vi "TXRX 5785 No DDC Measure Phase Stability_AI AO TCLK.vi"() -> ()   [LabVIEW 2019]
uses:
  <vilib>/userDefined/High Color/nirio_resource_hc.ctl
  <instrlib>/FlexRIO/API/Host/v1/NI FlexRIO/API/Reference Clock Source.ctl
  <vilib>/Analysis/1siggen.llb/Ramp Pattern by Delta.vi
  <instrlib>/FlexRIO/API/Host/v1/NI FlexRIO/API/Configure Reference Clock.vi
  <instrlib>/FlexRIO/API/Host/v1/NI FlexRIO/API/Get Property Reference - Fpga Small.vi
  <instrlib>/FlexRIO/API/Host/v1/NI FlexRIO/API/Configure Immediate Start Trigger.vi
  <instrlib>/FlexRIO/API/Host/v1/NI FlexRIO/API/Configure Digital Edge Start Trigger.vi
  <instrlib>/FlexRIO/API/Host/v1/NI FlexRIO/API/Read Stream 1D WDT.vi
  <vilib>/measure/matone.llb/Extract Single Tone Information N Chan.vi
  <vilib>/FPGAPlugInAG/Dynamic/niLvFpga_Close_Dynamic.vi
  <vilib>/Utility/file.llb/Write Delimited Spreadsheet (DBL).vi
  <vilib>/rvi/interface/nirviCloseFPGA/nirviCloseFPGA.xnode
  <vilib>/measure/NI_MAPro.lvlib
  <vilib>/Analysis/NI_AALPro.lvlib
  <vilib>/Analysis/NI_AALBase.lvlib
  <instrlib>/FlexRIO/API/Host/v1/NI FlexRIO API v1.lvlib
  <resource>/objmgr/niflexrioapiStream.rc
  Common/Original 5785 Example/Host/GettingStarted_5785_Host.lvlib
  <resource>/objmgr/niflexrioapiTrigger.rc
panel:
  out "read data 2":waveform(dbl)[](graph)=[{"t0"=timestamp(0 s since 1904-01-01), "dt"=3.125e-10, "Y"=[]}, {"t0"=timestamp(0 s since 1904-01-01), "dt"=3.125e-10, "Y"=[]}, {"t0"=timestamp(0 s since 1904-01-01), "dt"=3.125e-10, "Y"=[]}, {"t0"=timestamp(0 s since 1904-01-01), "dt"=3.125e-10, "Y"=[]}]
  in  "ABORT":bool
  in  "flexrio tranceivers":T2(array[cluster])
  out "error out":errorcluster
  out "read data":waveform(dbl)[](graph)=[{"t0"=timestamp(0 s since 1904-01-01), "dt"=3.125e-10, "Y"=[]}, {"t0"=timestamp(0 s since 1904-01-01), "dt"=3.125e-10, "Y"=[]}, {"t0"=timestamp(0 s since 1904-01-01), "dt"=3.125e-10, "Y"=[]}, {"t0"=timestamp(0 s since 1904-01-01), "dt"=3.125e-10, "Y"=[]}]
  in  "samples to acquire":u64=65536
  out "Output Waveform":waveform(dbl)[](graph)
  in  "sampling info":cluster{"Fs":dbl, "#s":dbl}={"Fs"=3200000000.0, "#s"=1600.0}
  in  "amplitude":dbl=0.2 format="%#_13p"
  in  "frequency":dbl=32000000.0 format="%0.2p"
  in  "trigger mode":enum16{"Immediate", "Digital"}(ring)
  in  "trigger source":string(combo)
  out "error out 2":errorcluster
  out "Results":T3(array[cluster])=[{"frequency (Hz)"=10000000.0, "mean skew"=-8.648150356036804e-11, "skew std dev"=2.4099744101288974e-11, "skew pk-pk"=7.257205272197028e-11, "skews"=[-7.634263492782065e-11, -5.206006966613256e-11, -7.567203753755032e-11, -1.2206425690719055e-10, -8.304777374940357e-11, -1.0474159284040468e-10, -9.611917176930304e-11, -4.9492204185220274e-11, -9.19555565839358e-11, -1.1331973743671892e-10]}, {"frequency (Hz)"=50000000.0, "mean skew"=-3.785636387258172e-12, "skew std dev"=7.66796131206532e-12, "skew pk-pk"=2.0450056958183634e-11, "skews"=[-1.4356702041335054e-11, -1.6858595580753508e-11, 3.9640356991197555e-13, 2.1898804487920657e-12, 3.591461377430126e-12, 5.627769488312176e-13, 2.0778793414142268e-12, -9.498878640875245e-13, -2.082260920467761e-12, -1.242731915231749e-11]}, {"frequency (Hz)"=100000000.0, "mean skew"=2.9756926970137243e-12, "skew std dev"=4.126438485430937e-12, "skew pk-pk"=1.3178656356672357e-11, "skews"=[-3.803864807523877e-12, 1.2229613162477112e-12, 3.353001868594509e-13, 6.147451569656316e-12, 3.467389040439413e-12, 9.37479154914848e-12, 3.130954906117878e-13, 5.3691066005407156e-12, 7.679194212684065e-12, -3.484981885268205e-13]}, {"frequency (Hz)"=150000000.0, "mean skew"=-3.1256285003637117e-12, "skew std dev"=2.50792505062644e-12, "skew pk-pk"=8.984925023293429e-12, "skews"=[-4.502762861812405e-12, -1.6045172273490561e-12, -2.9190171390647476e-12, -3.070990694678064e-13, -8.33215064320321e-12, -4.242400597204465e-12, -4.000839777166906e-12, 6.527743800902194e-13, -3.7005805394824356e-12, -2.2996915289763056e-12]}, {"frequency (Hz)"=200000000.0, "mean skew"=-8.350958023237677e-12, "skew std dev"=2.5975389756296594e-12, "skew pk-pk"=9.251979822405072e-12, "skews"=[-8.992508817543144e-12, -7.361526314260884e-12, -5.409418265633645e-12, -6.808722347470321e-12, -7.136097246425896e-12, -1.4661398088038717e-11, -1.0459370862648973e-11, -7.417267998914027e-12, -8.20329760295492e-12, -7.05997268848624e-12]}, {"frequency (Hz)"=250000000.0, "mean skew"=-6.229423609785982e-12, "skew std dev"=1.1181109842334413e-12, "skew pk-pk"=3.697563683201574e-12, "skews"=[-6.543472598258066e-12, -6.423877782336823e-12, -7.33916505767155e-12, -5.048427489200302e-12, -6.3111029457941555e-12, -6.605254632098134e-12, -6.962233060771497e-12, -3.95708736948471e-12, -5.448964109558302e-12, -7.654651052686284e-12]}, {"frequency (Hz)"=300000000.0, "mean skew"=-6.136089114075028e-12, "skew std dev"=9.42262857424596e-13, "skew pk-pk"=3.206385053636777e-12, "skews"=[-7.001117375279714e-12, -5.596228282724161e-12, -7.790788409887583e-12, -6.640956435014748e-12, -6.510029213872093e-12, -4.584403356250806e-12, -5.788671870420912e-12, -5.481861597872109e-12, -6.621852735719958e-12, -5.3449818637081885e-12]}, {"frequency (Hz)"=350000000.0, "mean skew"=-7.543098180047223e-12, "skew std dev"=3.8486735494540495e-13, "skew pk-pk"=1.2874637805991694e-12, "skews"=[-7.488662007824413e-12, -7.345064850347847e-12, -7.363173973336141e-12, -7.991225504656965e-12, -7.35831616172544e-12, -8.080201975318365e-12, -7.949579206730948e-12, -7.588239975011586e-12, -6.7927381947191955e-12, -7.473779950801325e-12]}, {"frequency (Hz)"=400000000.0, "mean skew"=-8.039336411333349e-12, "skew std dev"=7.425609882339821e-13, "skew pk-pk"=2.2738072930854095e-12, "skews"=[-7.656827769683663e-12, -9.457825738470782e-12, -7.679147937131138e-12, -7.995928800206408e-12, -8.83385230395903e-12, -7.54257226646767e-12, -7.31361750761873e-12, -7.184018445385372e-12, -7.962031171009181e-12, -8.767542173401512e-12]}, {"frequency (Hz)"=450000000.0, "mean skew"=-7.93200988579298e-12, "skew std dev"=7.97455496904726e-13, "skew pk-pk"=2.6238656725690157e-12, "skews"=[-7.898237136846618e-12, -8.55120393482239e-12, -8.79911402833156e-12, -7.812476697854857e-12, -7.693964239880247e-12, -6.482757646206027e-12, -8.3933125130091e-12, -9.106623318775042e-12, -7.260055680055343e-12, -7.322353662148608e-12]}, {"frequency (Hz)"=500000000.0, "mean skew"=-7.67982756908766e-12, "skew std dev"=6.672272359581462e-13, "skew pk-pk"=2.0371763701039724e-12, "skews"=[-8.507074422893644e-12, -7.0880582107488455e-12, -7.782804612094616e-12, -7.582126885479152e-12, -7.256810103118096e-12, -8.96121612129985e-12, -7.2605372159962215e-12, -7.281199578354681e-12, -6.924039751195878e-12, -8.154408789695609e-12]}, {"frequency (Hz)"=550000000.0, "mean skew"=-7.497637800191673e-12, "skew std dev"=7.103834430343908e-13, "skew pk-pk"=2.273387428636986e-12, "skews"=[-6.788566760330353e-12, -7.618981619747259e-12, -8.146972324445106e-12, -7.622320471598431e-12, -6.408580300349553e-12, -7.095092352672633e-12, -7.963135085088087e-12, -8.681967728986539e-12, -7.854698807254544e-12, -6.796062551444227e-12]}, {"frequency (Hz)"=600000000.0, "mean skew"=-6.656473926831814e-12, "skew std dev"=6.694881342261218e-13, "skew pk-pk"=1.9961300493555487e-12, "skews"=[-5.544977406952426e-12, -7.505826199727893e-12, -6.130703962050041e-12, -6.202863013065509e-12, -6.968667303110993e-12, -7.203039184312062e-12, -6.6392992458656125e-12, -6.0278794692841194e-12, -6.800376027641509e-12, -7.541107456307974e-12]}, {"frequency (Hz)"=650000000.0, "mean skew"=-6.170836312403341e-12, "skew std dev"=6.619061413781283e-13, "skew pk-pk"=2.2437727341724404e-12, "skews"=[-5.6761371841019825e-12, -6.355813112635683e-12, -5.813528117360099e-12, -5.8323315333927895e-12, -6.992345927519065e-12, -6.404883995266873e-12, -6.792134783464002e-12, -6.572966737937676e-12, -4.7485731933466245e-12, -6.5196485390086175e-12]}, {"frequency (Hz)"=700000000.0, "mean skew"=-6.189182831668323e-12, "skew std dev"=1.7157996931343636e-13, "skew pk-pk"=5.374178601958277e-13, "skews"=[-6.141615985942628e-12, -6.4858404095071854e-12, -6.233773633306086e-12, -6.2514132085703466e-12, -5.98652075251154e-12, -6.120870770642584e-12, -6.325272720314335e-12, -5.948422549311358e-12, -6.046719279911735e-12, -6.351379006665432e-12]}, {"frequency (Hz)"=750000000.0, "mean skew"=-6.5871572160487534e-12, "skew std dev"=4.41835545476434e-13, "skew pk-pk"=1.3482286990633495e-12, "skews"=[-6.408185337335485e-12, -6.6984014567953855e-12, -5.8037511563193215e-12, -5.956322167651966e-12, -6.385471028720583e-12, -7.009944685195322e-12, -6.796395481232521e-12, -6.839548682157055e-12, -6.821572309697221e-12, -7.151979855382671e-12]}, {"frequency (Hz)"=800000000.0, "mean skew"=-6.318415408299373e-12, "skew std dev"=5.360678898648873e-13, "skew pk-pk"=1.3845512042933417e-12, "skews"=[-6.991605843987897e-12, -6.471917002931961e-12, -5.868508226304447e-12, -6.587798178445769e-12, -5.6267669909771774e-12, -6.078767737351072e-12, -5.619707707506443e-12, -7.0042589117997844e-12, -6.851992861208232e-12, -6.082830622480952e-12]}, {"frequency (Hz)"=850000000.0, "mean skew"=-6.0180248346099665e-12, "skew std dev"=3.591713662163337e-13, "skew pk-pk"=1.1349470370084415e-12, "skews"=[-5.778738385130886e-12, -5.507329414754426e-12, -6.00610567960471e-12, -6.351181258112003e-12, -6.642276451762867e-12, -6.120739453272636e-12, -5.830550574804746e-12, -6.130742822105978e-12, -6.26599539616416e-12, -5.5465889103872445e-12]}, {"frequency (Hz)"=900000000.0, "mean skew"=-6.105366074378527e-12, "skew std dev"=2.6415729684293626e-13, "skew pk-pk"=9.150989335434855e-13, "skews"=[-6.100624138292147e-12, -6.176574316377945e-12, -6.247087188419655e-12, -6.696716487837525e-12, -5.835346835163569e-12, -5.994420432808338e-12, -6.201485877561482e-12, -5.78161755429404e-12, -5.8764077856967975e-12, -6.143380127333783e-12]}, {"frequency (Hz)"=950000000.0, "mean skew"=-6.431589636547766e-12, "skew std dev"=2.1126924807836585e-13, "skew pk-pk"=6.684732217835237e-13, "skews"=[-6.4527930268702555e-12, -6.67300399028584e-12, -6.020076613990734e-12, -6.561072065807103e-12, -6.250560131333176e-12, -6.440878292553848e-12, -6.404316276846632e-12, -6.580400983912426e-12, -6.244245148103377e-12, -6.6885498357742574e-12]}, {"frequency (Hz)"=1000000000.0, "mean skew"=-6.675839066411157e-12, "skew std dev"=3.266749368738765e-13, "skew pk-pk"=9.515417562958724e-13, "skews"=[-6.645668230188316e-12, -7.064422435097906e-12, -6.696684468644875e-12, -6.525650475721844e-12, -7.024648721850936e-12, -6.648717189793257e-12, -7.15475948867288e-12, -6.563526021551009e-12, -6.231095900213532e-12, -6.203217732377007e-12]}] {"frequency (Hz)" format="%#_6p"; "mean skew" format="%#_6p"; "skew std dev" format="%#_6p"; "skew pk-pk" format="%#_6p"; "skews" format="%#_6p"}
  out "Current Frequency Under Test":dbl=1000000000.0 format="%#_6p"
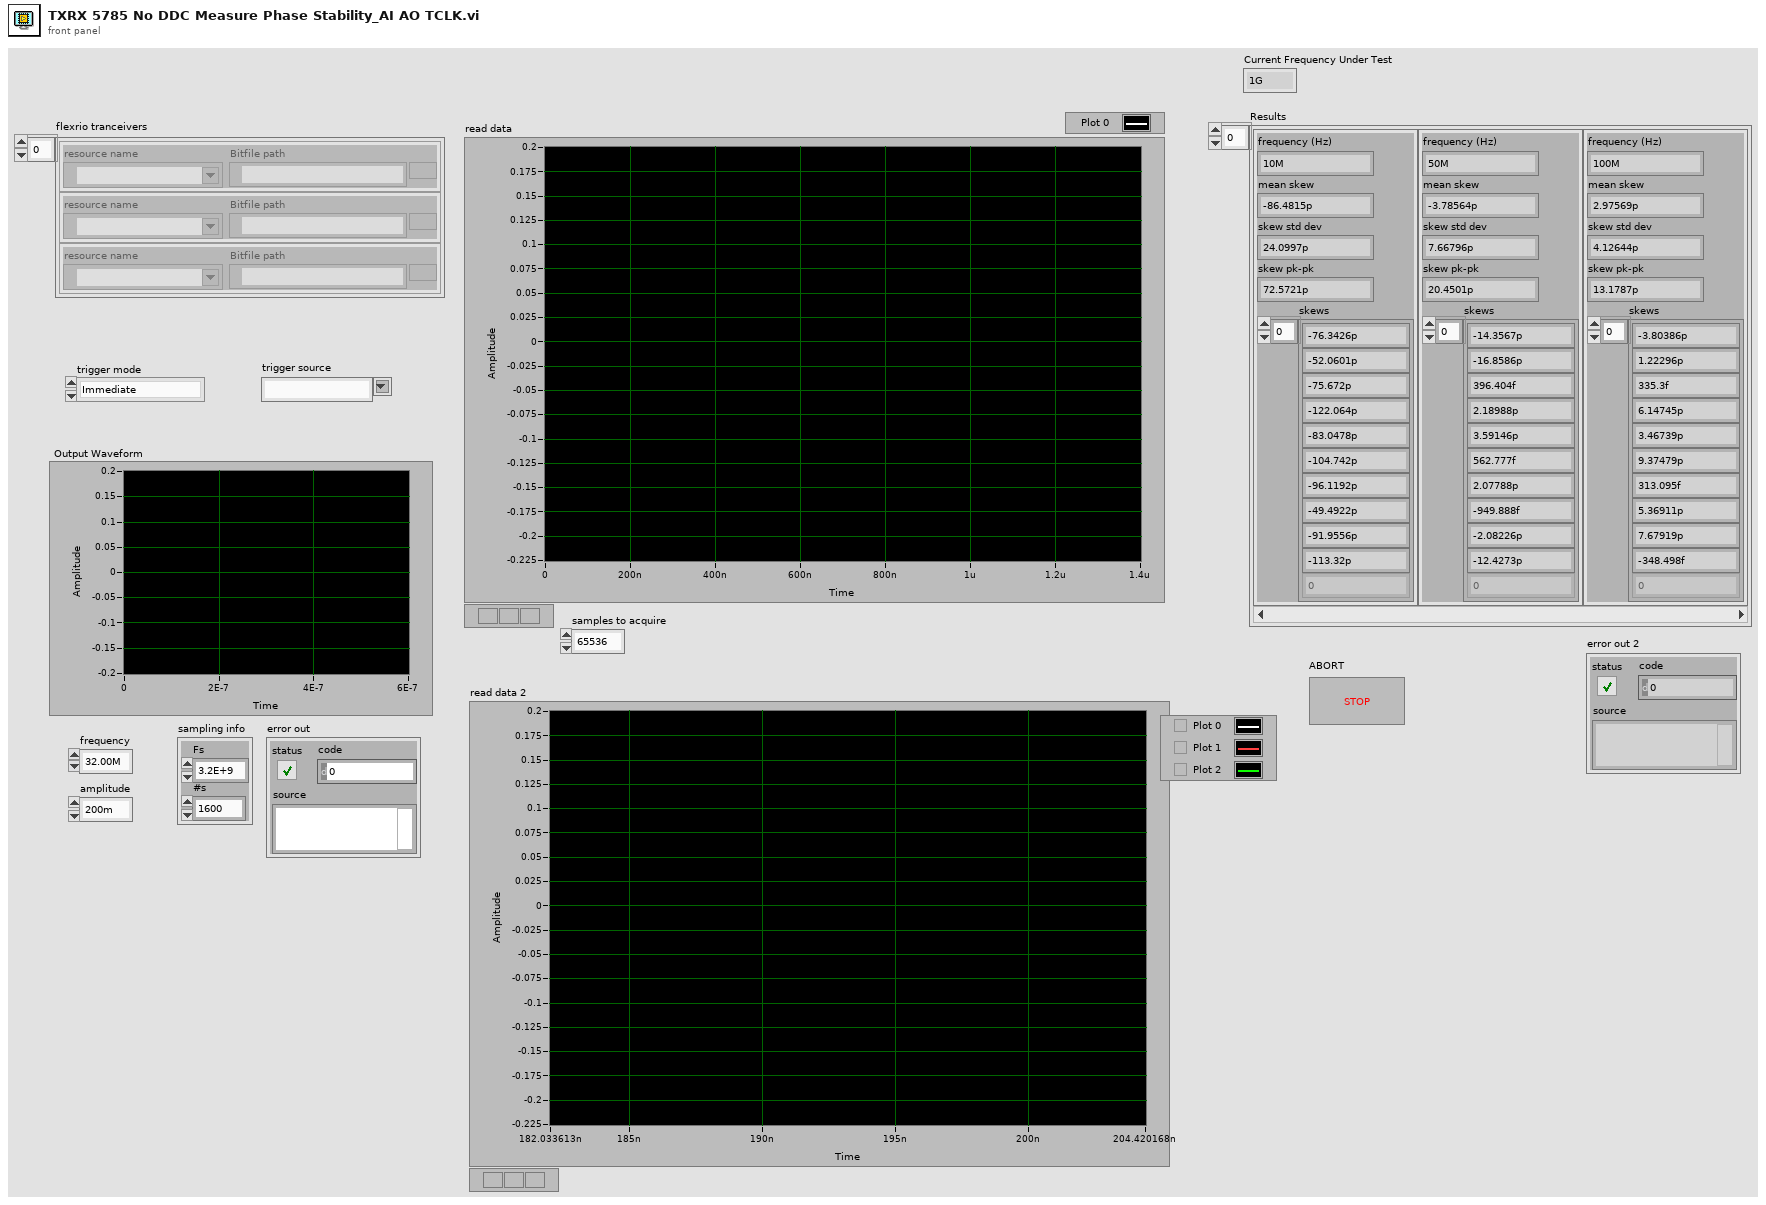
[diagram p1: front panel]
types:
  T1 = typedef "nirio_resource_hc.ctl" = tag
  T2 = cluster{"resource name":T1, "Bitfile path":path}[]
  T3 = cluster{"frequency (Hz)":dbl, "mean skew":dbl, "skew std dev":dbl, "skew pk-pk":dbl, "skews":dbl[]}[]
  T4 = cluster{"frequency":dbl, "mean skew":dbl, "skew std dev":dbl, "skew pk-pk":dbl, "skews":dbl[]}
  T5 = typedef "NI FlexRIO API v1.lvlib/Reference Clock Source.ctl" = i32
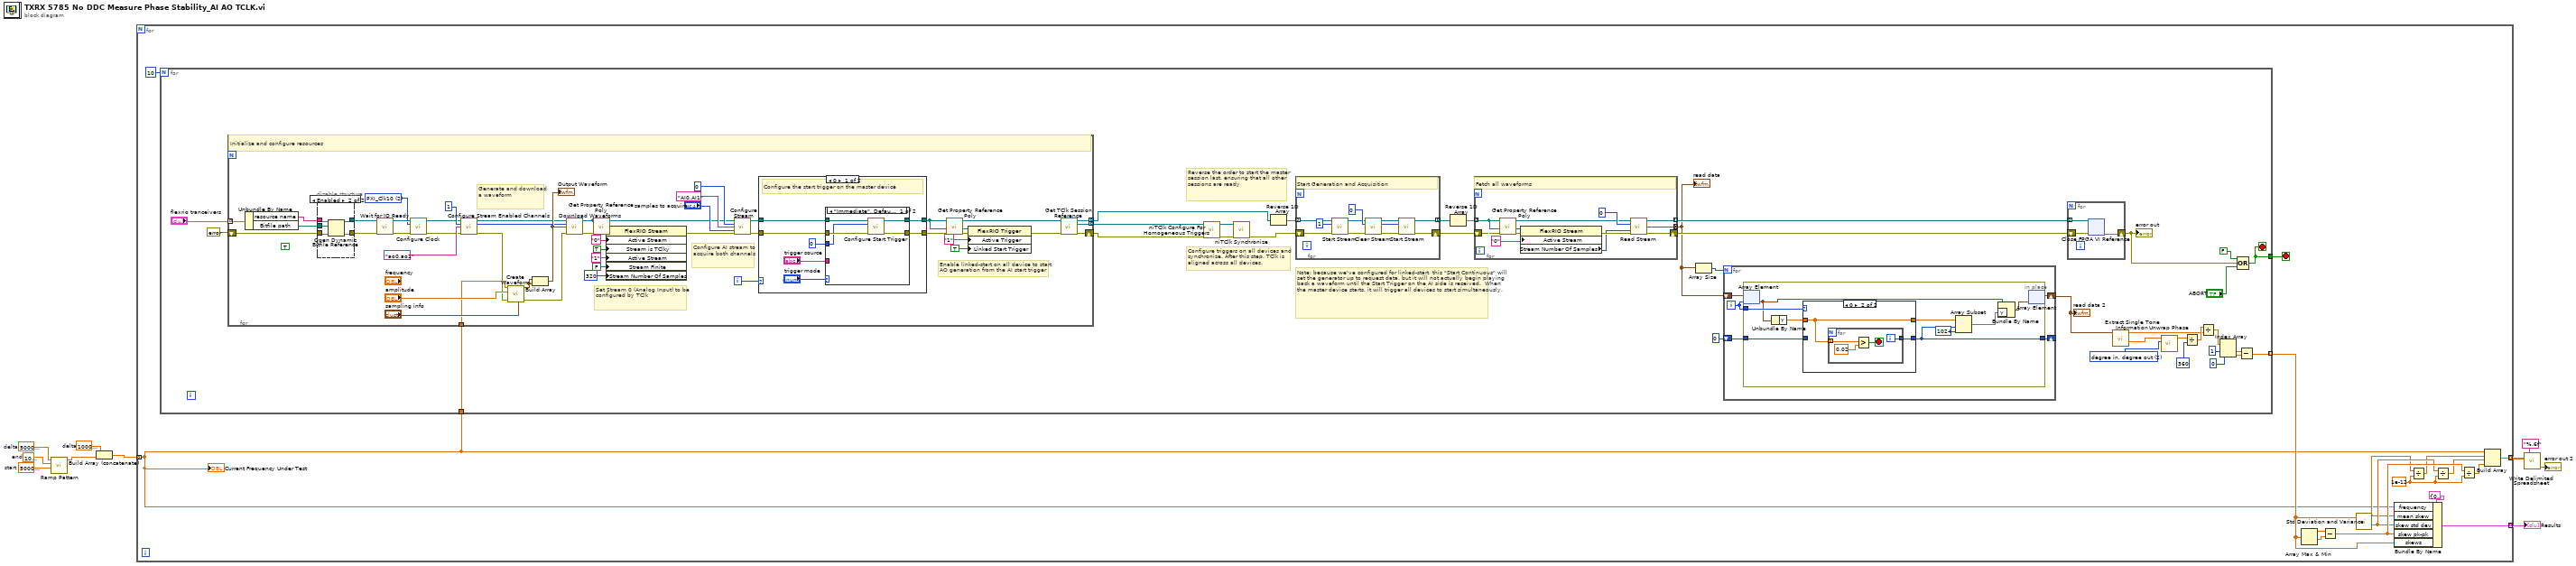
[diagram p0: block diagram]
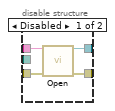
[diagram p3: hidden frame]
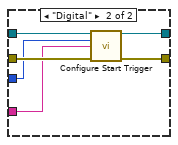
[diagram p4: hidden frame]
diagram:
  w3 = 10000000.0  # delta
  w8 = 50000000.0  # delta
  w9 = 1000000000.0  # end
  w10 = 50000000.0  # start
  n1 = call-poly <vilib>:"Ramp Pattern.vi"("start"=w10, "end"=w9, "delta"=w8) -> ("Ramp Pattern"=w7:dbl[])  [unwired: 6 in, 2 out]
  n2 = Build Array (concatenate)(w3, w7) -> (w4:dbl[])
  n3 = for {
    tunnel: [w15] -> w6 mode=indexing
    tunnel: [w14] -> w5 mode=indexing
    tunnel: w4 -> [w12] mode=indexing
    stop <- w11 stop-if-true
    w16 = 1e-12 ("y")
    n4 = for {
      N: 10 -> [_]
      tunnel: [w51] -> w13 mode=indexing
      tunnel: w12 -> [w33]
      tunnel: [w36] -> w11
      stop <- w36 stop-if-true
      w57 = 2 items=["radian in, radian out", "radian in, degree out", "degree in, degree out", "degree in, radian out"] ("phase unit")
      # "Note: because we've configured for linked-start, this \"Start Continuous\" will set the generator up to request data, but it will not actually begin playing back a waveform until the Start Trigger on the AI side is received.  When the master device starts, it will trigger all devices to start simultaneously."
      # "Reverse the order to start the master session last, ensuring that all other sessions are ready"
      # "Configure triggers on all devices and\nsynchronize. After this step, TClk is\naligned across all devices."
      n5 = for {
        shift-right: [w137] -> w38
        shift-left: errorcluster {"status"=FALSE, "code"=0, "source"=""} ("error out") -> [w112]
        tunnel: "flexrio tranceivers" -> [w142] mode=indexing
        tunnel: [w136] -> w39 mode=indexing
        tunnel: [w135] -> w37 mode=indexing
        tunnel: w33 -> [w109]
        i -> [w138]
        w118 = T5 2 items=["Default", "Onboard", "PXI_Clk10", "External", "None", "Baseboard Reference"] ("reference clock source")
        (unwired) TRUE ("Run When Loaded")
        # "Enable linked-start on all device to start\nAO generation from the AI start trigger"
        # "Configure AI stream to acquire both channels"
        # "Set Stream 0 (Analog Input) to be configured by TClk"
        # "Generate and download a waveform"
        # "Initialize and configure resources"
        n6 = Unbundle By Name(w142) -> ("resource name"=w111:T1, "Bitfile path"=w110:path)
        n7 = disable-structure shown="Enabled" {
          disable-tunnel: [w160 w164] -> w114
          disable-tunnel: [w159 w165] -> w113
          disable-tunnel: w112 -> [w158 w161]
          disable-tunnel: w111 -> [w157 w163]
          disable-tunnel: w110 -> [_ w162]
          frame Disabled {
            n8 = call <instrlib>:"Open.vi"("RIO Device"=w157, "error in"=w158) -> ("fpga interface out"=w160:refnum<k20>, "error out"=w159:errorcluster)  [unwired: 12 in]
          }
          frame Enabled {
            n9 = Open Dynamic Bitfile Reference(0:w163, 1:w162, 3:w161) -> (5:w164:refnum<k20>, 8:w165:errorcluster)  [unwired: 2 in]
          }
        }
        n10 = call <instrlib>:"Wait for IO Ready.vi"("fpga interface in"=w114, "error in"=w113) -> ("fpga interface out"=w122:refnum<k20>, "error out"=w119:errorcluster)  [unwired: 10 in, 2 out]
        n11 = call-poly <instrlib>:"Configure Clock.vi"("fpga interface in"=w122, "reference clock source"=w118, "error in"=w119) -> ("fpga interface out"=w121:refnum<k20>, "error out"=w120:errorcluster)  [unwired: 11 in]
        n12 = call <instrlib>:"Configure Stream Enabled Channels.vi"("fpga interface in"=w121, "stream instance"=u32 1, "channels enabled"="ao0,ao1", "error in"=w120) -> ("fpga interface out"=w127:refnum<k20>, "stream instance out"=w123:u32, "error out"=w126:errorcluster)  [unwired: 8 in, 1 out]
        n13 = call "Create Waveform.vi"("sampling info"="sampling info", "error in (no error)"=w126, "amplitude"="amplitude", "frequency"=w109) -> ("error out"=w141:errorcluster, "Output Waveform (V)"=w146:waveform(dbl))  [unwired: 5 in, 1 out]
        n14 = Build Array(w146, w146) -> (w144:waveform(dbl)[])
        "Output Waveform" <- w144
        n15 = call "Download Waveforms.vi"("fpga interface in"=w127, "stream instance"=w123, "waveforms"=w144, "error in"=w141) -> ("fpga interface out"=w145:refnum<k20>, "error out"=w143:errorcluster)  [unwired: 9 in, 1 out]
        n16 = call-poly <instrlib>:"Get Property Reference Poly.vi"("error in (no error)"=w143, "fpga interface in"=w145) -> ("error out"=w156:errorcluster, "property reference"=w155:refnum<k20>)  [unwired: 4 in, 1 out]
        n17 = property class="FlexRIO Stream"(reference=w155, error in=w156, "Active Stream"="0", "Stream is TClky"=TRUE ("Configuration:Stream is TClky"), "Active Stream"="1", "Stream Finite"=FALSE ("Configuration:Finite"), "Stream Number Of Samples"=u64 320) -> (error out=w152:errorcluster)  [unwired: 1 out]
        n18 = call <instrlib>:"Configure Stream.vi"("fpga interface in"=w145, "stream instance"=u32 0, "channels enabled"="AI0,AI1", "num samples"="samples to acquire", "error in"=w152) -> ("fpga interface out"=w140:refnum<k20>, "error out"=w139:errorcluster)  [unwired: 7 in, 2 out]
        n19 = case shown="0" w138 {
          tunnel: [w170 w185] -> w128
          tunnel: w140 -> [w169 w185]
          tunnel: w139 -> [w168 w184]
          tunnel: [w167 w184] -> w131
          frame 0 {
            # "Configure the start trigger on the master device"
            n20 = case shown="\"Immediate\", Default" "trigger mode" {
              tunnel: w168 -> [w177 w182]
              tunnel: w169 -> [w174 w183]
              tunnel: [w176 w181] -> w167
              tunnel: [w173 w180] -> w170
              tunnel: u32 0 ("trigger instance") -> [w175 w179]
              tunnel: "trigger source" -> [_ w178]
              frame "Immediate", Default {
                n21 = call-poly <instrlib>:"Configure Start Trigger.vi"("fpga interface in"=w174, "trigger instance"=w175, "error in"=w177) -> ("fpga interface out"=w173:refnum<k20>, "error out"=w176:errorcluster)  [unwired: 10 in, 1 out]
              }
              frame "Digital" {
                n22 = call-poly <instrlib>:"Configure Start Trigger.vi"("fpga interface in"=w183, "trigger instance"=w179, "trigger source"=w178, "error in"=w182) -> ("fpga interface out"=w180:refnum<k20>, "error out"=w181:errorcluster)  [unwired: 9 in, 1 out]
              }
            }
          }
          frame 1, Default {
            # "Do not configure a trigger on the slaves (TClk will)"
          }
        }
        n23 = call-poly <instrlib>:"Get Property Reference Poly.vi"("error in (no error)"=w131, "fpga interface in"=w128) -> ("error out"=w134:errorcluster, "property reference"=w133:refnum<k20>)  [unwired: 4 in, 1 out]
        n24 = property class="FlexRIO Trigger"(reference=w133, error in=w134, "Active Trigger"="1" ("Active Stream"), "Linked Start Trigger"=TRUE ("Start:Linked")) -> (error out=w129:errorcluster)  [unwired: 1 out]
        n25 = call <instrlib>:"Get TClk Session Reference.vi"("fpga interface in"=w128, "error in"=w129) -> ("fpga interface out"=w136:refnum<k20>, "tclk session reference"=w135:refnum<k20>, "error out"=w137:errorcluster)  [unwired: 11 in]
      }
      n26 = call <instrlib>:"niTClk Configure For Homogeneous Triggers.vi"("error in (no error)"=w38, "sessions"=w37) -> ("error out"=w50:errorcluster, "sessions out"=w49:refnum<k20>[])  [unwired: 8 in]
      n27 = call <instrlib>:"niTClk Synchronize.vi"("error in (no error)"=w50, "sessions"=w49) -> ("error out"=w47:errorcluster)  [unwired: 8 in, 1 out]
      n28 = Reverse 1D Array(array=w39) -> (reversed array=w48:refnum<k20>[])
      n29 = for {
        tunnel: w48 -> [w102] mode=indexing
        shift-right: [w108] -> w45
        shift-left: w47 -> [w101]
        tunnel: [w107] -> w46 mode=indexing
        # "Start Generation and Acquisition"
        n30 = call <instrlib>:"Start Stream.vi"("fpga interface in"=w102, "stream instance"=u32 1, "error in"=w101) -> ("fpga interface out"=w99:refnum<k20>, "error out"=w98:errorcluster)  [unwired: 10 in, 1 out]
        n31 = call <instrlib>:"Clear Stream.vi"("fpga interface in"=w99, "stream instance"=u32 0, "error in"=w98) -> ("fpga interface out"=w105:refnum<k20>, "stream instance out"=w103:u32, "error out"=w106:errorcluster)  [unwired: 10 in]
        n32 = call <instrlib>:"Start Stream.vi"("fpga interface in"=w105, "stream instance"=w103, "error in"=w106) -> ("fpga interface out"=w107:refnum<k20>, "error out"=w108:errorcluster)  [unwired: 10 in, 1 out]
      }
      n33 = Reverse 1D Array(array=w46) -> (reversed array=w44:refnum<k20>[])
      n34 = for {
        tunnel: w44 -> [w87] mode=indexing
        tunnel: [w90] -> w30 mode=concatenating
        shift-right: [w89] -> w42
        shift-left: w45 -> [w94]
        tunnel: [w88] -> w43 mode=indexing
        # "Fetch all waveforms"
        n35 = call-poly <instrlib>:"Get Property Reference Poly.vi"("error in (no error)"=w94, "fpga interface in"=w87) -> ("error out"=w97:errorcluster, "property reference"=w96:refnum<k20>)  [unwired: 4 in, 1 out]
        n36 = property class="FlexRIO Stream"(reference=w96, error in=w97, "Active Stream"="0") -> (error out=w93:errorcluster, "Stream Number Of Samples"=w92:u64)  [unwired: 1 out]
        n37 = call-poly <instrlib>:"Read Stream.vi"("fpga interface in"=w87, "stream instance"=u32 0, "samples"=w92, "error in"=w93) -> ("fpga interface out"=w88:refnum<k20>, "read data"=w90:waveform(dbl)[], "error out"=w89:errorcluster)  [unwired: 7 in, 2 out]
      }
      "read data" <- w30
      n38 = Array Size(array=w30) -> (size(s)=w32:i32)
      n39 = for {
        N: w32 -> [_]
        shift-right: [w63] -> _
        shift-left: 0 -> [w62]
        shift-right: [w65] -> w29
        shift-left: w30 -> [w66]
        i -> [w64]
        n40 = in-place {
          in-place-border: w64 -> [w75]
          in-place-border: [w71] -> w63
          in-place-border: w62 -> [w73]
          n41 = in-place-array #1(w66, w64) -> (w69:waveform(dbl))
          n42 = Unbundle By Name(w69) -> ("Y"=w74:dbl[])
          n43 = case shown="0" w75 {
            tunnel: w74 -> [w77 w79]
            tunnel: [w77 w79] -> w72
            tunnel: [w76 w78] -> w71
            tunnel: w73 -> [w76 _]
            frame 1.., Default {
            }
            frame 0 {
              n44 = for {
                tunnel: w79 -> [w83] mode=indexing
                tunnel: [w80] -> w78
                i -> [w80]
                stop <- w82 stop-if-true
                n45 = Greater?(x=w83, y=0.02) -> (0:w82:bool)
              }
            }
          }
          n46 = Array Subset(array=w72, index=w71, length=1024) -> (w68:dbl[])
          n47 = Bundle By Name(cluster=w69, "Y"=w68) -> (w67:waveform(dbl))
          n48 = in-place-array #1(w67) -> (w65:waveform(dbl)[])  [unwired: 1 out]
        }
      }
      "read data 2" <- w29
      n49 = for {
        tunnel: w43 -> [w85] mode=indexing
        shift-right: [w84] -> w35
        shift-left: w42 -> [w86]
        n50 = xnode "Close FPGA VI Reference"("FPGA VI Reference In"=w85, "error in"=w86) -> ("error out"=w84:errorcluster)
      }
      "error out" <- w35
      n51 = call-poly <vilib>:"Extract Single Tone Information.vi"("time signals in"=w29) -> ("detected phases (deg)"=w27:dbl[], "detected frequencies"=w52:dbl[])  [unwired: 5 in, 4 out]
      n52 = call <vilib>:"Unwrap Phase.vi"("phase unit"=w57, "Phase"=w27) -> ("Unwrapped Phase"=w61:dbl[])  [unwired: 8 in, 1 out]
      n53 = Divide(x=w61, y=360) -> (x/y=w60:dbl[])
      n54 = Divide(x=w60, y=w52) -> (x/y=w58:dbl[])
      n55 = Index Array(array=w58, index #1=1 ("index (row)"), index #2=0 ("index (row)")) -> (element #1=w54:dbl, element #2=w53:dbl)
      n56 = Compound Arithmetic op=OR(FALSE, w35, "ABORT") -> (w36:bool)
      n57 = Subtract(x=w54, y=w53) -> (x-y=w51:dbl)
    }
    n58 = Array Max & Min(array=w13) -> (max value=w19:dbl, min value=w18:dbl)  [unwired: 2 out]
    n59 = Subtract(x=w19, y=w18) -> (x-y=w24:dbl)
    n60 = call <vilib>:"Std Deviation and Variance.vi"("X"=w13) -> ("mean"=w20:dbl, "standard deviation"=w22:dbl)  [unwired: 1 in, 1 out]
    n61 = Bundle By Name(cluster=T4 {"frequency"=0.0, "mean skew"=0.0, "skew std dev"=0.0, "skew pk-pk"=0.0, "skews"=[]}, "frequency"=w12, "mean skew"=w20, "skew std dev"=w22, "skew pk-pk"=w24, "skews"=w13) -> (w14:T4)
    n62 = Divide(x=w20, y=w16) -> (x/y=w21:dbl)
    n63 = Divide(x=w22, y=w16) -> (x/y=w23:dbl)
    n64 = Divide(x=w24, y=w16) -> (x/y=w25:dbl)
    n65 = Build Array(w12, w21, w23, w25) -> (w15:dbl[])
    "Current Frequency Under Test" <- w12
  }
  "Results" <- w5
  n66 = call-poly <vilib>:"Write Delimited Spreadsheet.vi"("format (%.3f)"="%.6f", "2D data"=w6) -> ("error out"=→"error out 2":errorcluster)  [unwired: 12 in, 1 out]
